vi "calculate R (CDB).vi"(10 "eigenvalue":cdb, 11 "Array":cdb[][][](array[numeric])) -> (3 "R":cdb[][](array[numeric]))   [LabVIEW 2020, in "NI_AALPro.lvlib"]
uses:
  <vilib>/Analysis/NI_AALPro.lvlib
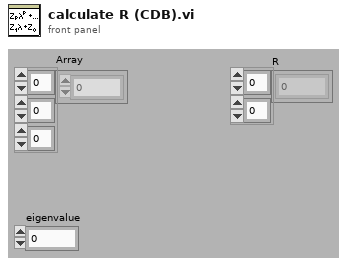
[diagram p1: front panel]
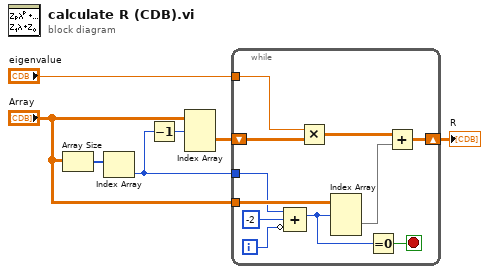
[diagram p0: block diagram]
diagram:
  n1 = Array Size(array="Array") -> (size(s)=w7:i32[])
  n2 = Index Array(array=w7) -> (element=w4:i32)  [unwired: 1 in]
  n3 = Decrement(x=w4) -> (x-1=w6:i32)
  n4 = Index Array(array="Array", index (dim 0)=w6) -> (element=w3:cdb[][])  [unwired: 2 in]
  n5 = while {
    tunnel: "Array" -> [w18]
    tunnel: w4 -> [w17]
    shift-right: [w8] -> w1
    shift-left: w3 -> [w11]
    tunnel: "eigenvalue" -> [w12]
    i -> [w16]
    stop <- w14 stop-if-true
    n6 = Compound Arithmetic op=ADD(w17, -2, invert w16) -> (w13:i32)
    n7 = Multiply(x=w12, y=w11) -> (x*y=w9:cdb[][])
    n8 = Index Array(array=w18, index (dim 0)=w13) -> (element=w10:cdb[][])  [unwired: 2 in]
    n9 = Equal To 0?(x=w13) -> (x = 0?=w14:bool)
    n10 = Add(x=w9, y=w10) -> (x+y=w8:cdb[][])
  }
  "R" <- w1
